vi "Check Trigger Source.vi"(0 "configured channels":bool[](array[boolean]), 5 "trigger source":u8, 11 "error in":errorcluster) -> (15 "error out":errorcluster)   [LabVIEW 2021, in "Device Session.lvclass"]
uses:
  Device Session.lvclass
  <vilib>/Utility/error.llb/Error Cluster From Error Code.vi
  <vilib>/ErrorRing/Error Ring.xnode
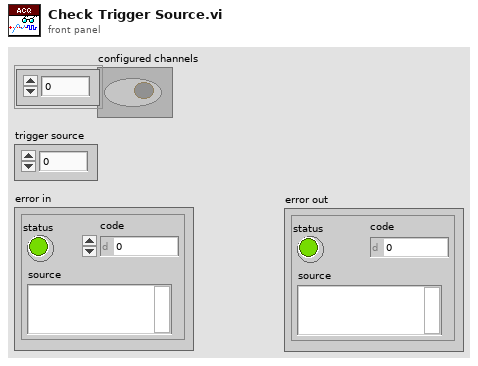
[diagram p1: front panel]
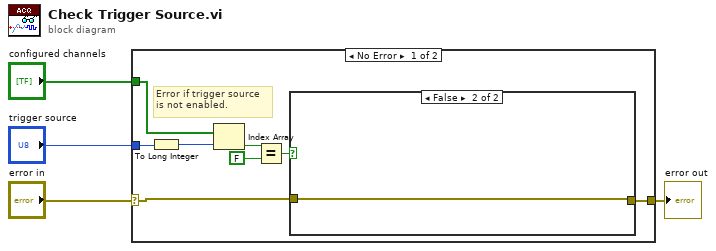
[diagram p0: block diagram]
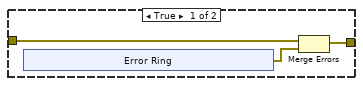
[diagram p2: hidden frame]
diagram:
  n1 = case shown="No Error" "error in" {
    selector: "error in" -> [w5 w21]
    tunnel: [w12 w21] -> w1
    tunnel: "configured channels" -> [w10 _]
    tunnel: "trigger source" -> [w7 _]
    frame No Error {
      # "Error if trigger source is not enabled."
      n2 = To Long Integer(number=w7) -> (32bit integer=w6:i32)
      n3 = Index Array(array=w10, index=w6) -> (element=w9:bool)
      n4 = Equal?(x=w9, y=FALSE) -> (x = y?=w8:bool)
      n5 = case shown="False" w8 {
        tunnel: [w13 w20] -> w12
        tunnel: w5 -> [w15 w20]
        frame True {
          n6 = xnode "Error Ring"() -> ("error out"=w14:errorcluster)
          n7 = Merge Errors(w15, w14) -> (w13:errorcluster)
        }
        frame False {
        }
      }
    }
    frame Error {
    }
  }
  "error out" <- w1
